vi "CAN Start Schedule.vi"(7 "MsgNum":u32, 9 "pCanMsg":T1, 10 "CANIndex":u8, 11 "DevHandle":i32) -> (1 "pCanMsg out":T1, 3 "function return":i32)   [LabVIEW 2010, in "usb2can.lvlib"]
doc: "int WINAPI CAN_StartSchedule(int DevHandle, unsigned char CANIndex, PCAN_MSG pCanMsg,unsigned int MsgNum);"
uses:
  usb2can.lvlib
  USB2XXX.dll
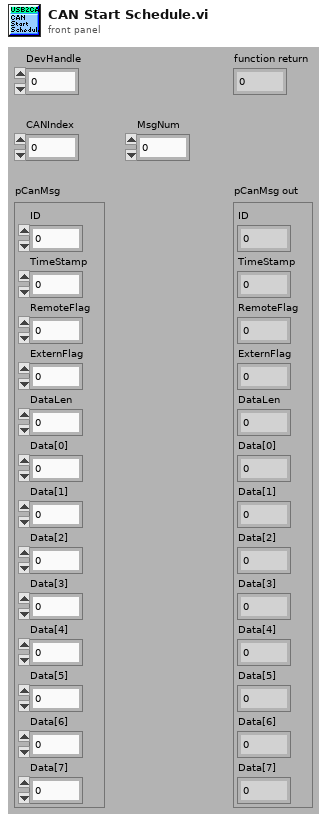
[diagram p1: front panel]
types:
  T1 = cluster{"ID":u32, "TimeStamp":u32, "RemoteFlag":u8, "ExternFlag":u8, "DataLen":u8, "Data[0]":u8, "Data[1]":u8, "Data[2]":u8, "Data[3]":u8, "Data[4]":u8, "Data[5]":u8, "Data[6]":u8, "Data[7]":u8}
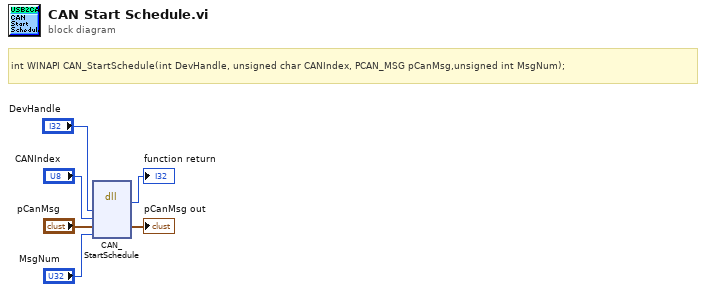
[diagram p0: block diagram]
diagram:
  # "int WINAPI CAN_StartSchedule(int DevHandle, unsigned char CANIndex, PCAN_MSG pCanMsg,unsigned int MsgNum);"
  n1 = dll-call lib="E:/OtherWork/STM32/USB2XXX_Example/sdk/api/Labview/USB2XXX.*" fn="CAN_StartSchedule"("DevHandle"="DevHandle", "CANIndex"="CANIndex", "pCanMsg"="pCanMsg", "MsgNum"="MsgNum") -> (→"function return":i32, "pCanMsg"=→"pCanMsg out":T1)  [unwired: 6 in, 2 out]
